vi "GetDisplays.vi"(8 "No Error":errorcluster) -> (0 "Error Out":errorcluster, 3 "Display IDs":T1[](array[typedef]))   [LabVIEW 2024, in "SDL3.lvlib" / "Video.lvlib"]
doc: "<B>Summary</B>\nGet a list of currently connected displays."
uses:
  Video.lvlib
  DisplayID--integer.ctl
  Error/Error.lvlib
  Stdinc/Stdinc.lvlib
  Lib/SDL3-32.dll
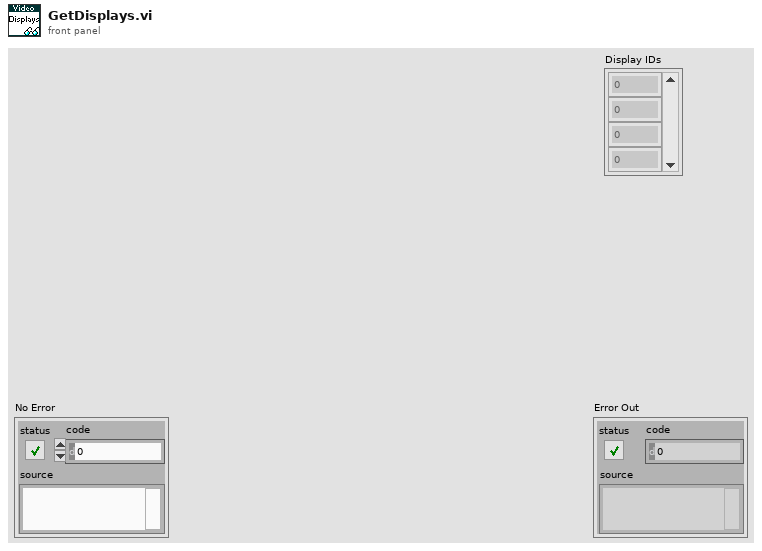
[diagram p1: front panel]
types:
  T1 = typedef "SDL3.lvlib/Video.lvlib/DisplayID--integer.ctl" = u32
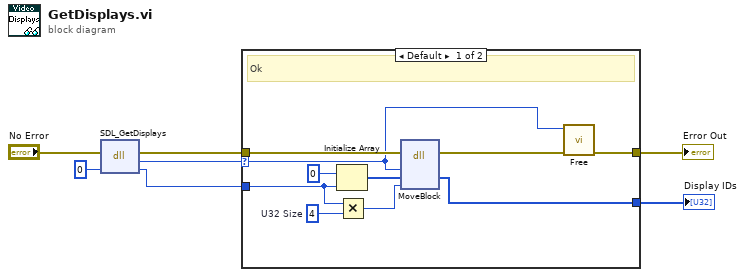
[diagram p0: block diagram]
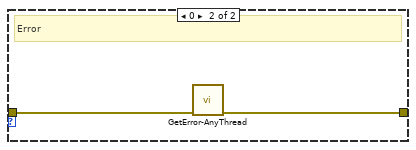
[diagram p2: hidden frame]
diagram:
  n1 = dll-call lib="C:/Users/Thomas/Documents/Projects/LV-SDL3/Lib/SDL3-*.*" fn="SDL_GetDisplays"(error in="No Error", "count"=0) -> (error out=w4:errorcluster, "return type"=w3:i64, "count"=w2:i32)  [unwired: 2 in, 1 out]
  n2 = case shown="Default" w3 {
    selector: w3 -> [w8 _]
    tunnel: w4 -> [w17 w19]
    tunnel: [w9 w18] -> w6
    tunnel: w2 -> [w12 _]
    tunnel: [w13 _] -> w1
    frame Default {
      w10 = 4  # U32 Size
      # "Ok"
      n3 = Initialize Array(T1 0 ("DisplayID"), w12) -> (w14:T1[])
      n4 = Multiply(x=w12, y=w10) -> (x*y=w11:i32)
      n5 = dll-call lib="LabVIEW" fn="MoveBlock"(error in=w17, "Address"=w8, "Destination"=w14, "Size"=w11) -> (error out=w16:errorcluster, "Destination"=w13:T1[])  [unwired: 5 in, 1 out]
      n6 = call "Free.vi"("No Error"=w16, "Mem [void *]"=w8) -> ("Error Out"=w9:errorcluster)  [unwired: 9 in]
    }
    frame 0 {
      # "Error"
      n7 = call "GetError-AnyThread.vi"("No Error"=w19) -> ("Error Out"=w18:errorcluster)  [unwired: 10 in]
    }
  }
  "Error Out" <- w6
  "Display IDs" <- w1
